vi "movement.vi"(4 "nextPos":cluster{"x":dbl, "y":dbl, "stop?":bool}, 5 "robotPos":cluster{"x":dbl, "y":dbl, "theta":dbl}) -> (0 "stop?":bool, 1 "arrived?":bool, 2 "outputSpeed":cluster{"left":dbl, "right":dbl}={"left"=1.0, "right"=-1.0})   [LabVIEW 2016]
panel:
  in  "input cluster":cluster{"x":dbl, "y":dbl}
  in  "distanceThreshold":dbl=100.0
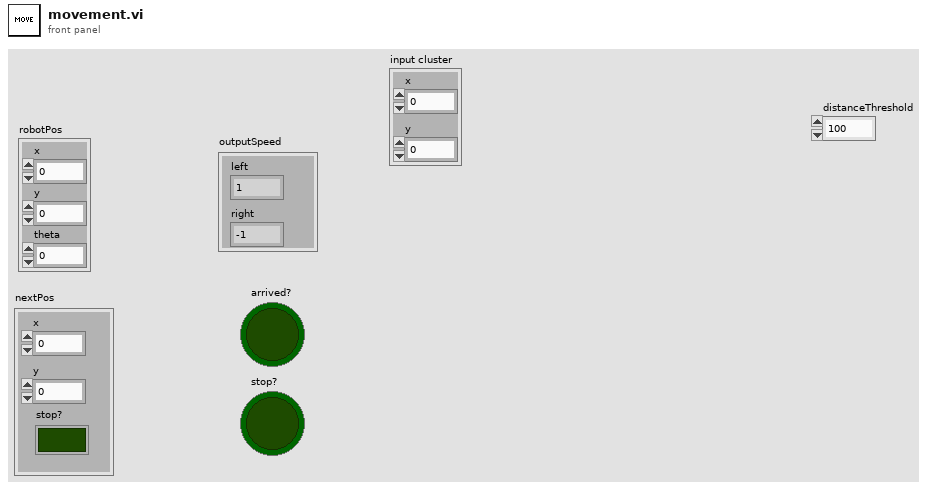
[diagram p1: front panel]
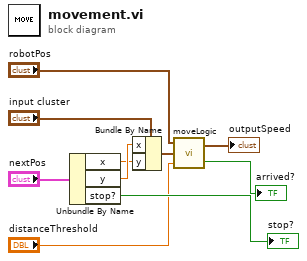
[diagram p0: block diagram]
diagram:
  n1 = Unbundle By Name("nextPos") -> ("x"=w1:dbl, "y"=w2:dbl, "stop?"=→"stop?":bool)
  n2 = Bundle By Name(cluster="input cluster", "x"=w2, "y"=w1) -> (w5:cluster{"x":dbl, "y":dbl})
  n3 = call "moveLogic.vi"("distanceThreshold"="distanceThreshold", "nextPos"=w5, "robotPos"="robotPos") -> ("arrived?"=→"arrived?":bool, "outputSpeed"=→"outputSpeed":cluster{"left":dbl, "right":dbl})
